vi "Drive PID.vi"(4 "reinitialize? (F)":bool, 6 "PID Params":T1={"PID gains"={"proportional gain (Kc)"=1.0, "integral time (Ti, min)"=0.0, "derivative time (Td, min)"=0.0}, "output range"={"output high"=1.0, "output low"=-1.0}}, 7 "Setpoint":dbl, 8 "Max Stop Speed":dbl, 9 "Distance Stop Threshold":dbl, 10 "Current Speed":dbl, 11 "Current Distance":dbl format="%#_13g") -> (0 "Finished":bool, 2 "output":dbl format="%.2f")   [LabVIEW 2014]
uses:
  <vilib>/addons/control/pid/pid.llb/PID (DBL).vi
  <vilib>/addons/control/pid/NI_PID_pid.lvlib
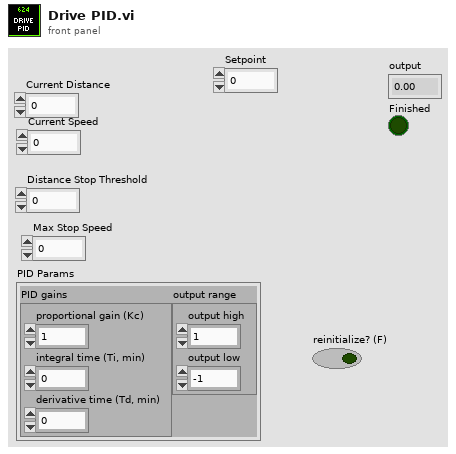
[diagram p1: front panel]
types:
  T1 = cluster{"PID gains":cluster{"proportional gain (Kc)":dbl, "integral time (Ti, min)":dbl, "derivative time (Td, min)":dbl}, "output range":cluster{"output high":dbl, "output low":dbl}}
  T2 = cluster{"proportional gain (Kc)":dbl, "integral time (Ti, min)":dbl, "derivative time (Td, min)":dbl}
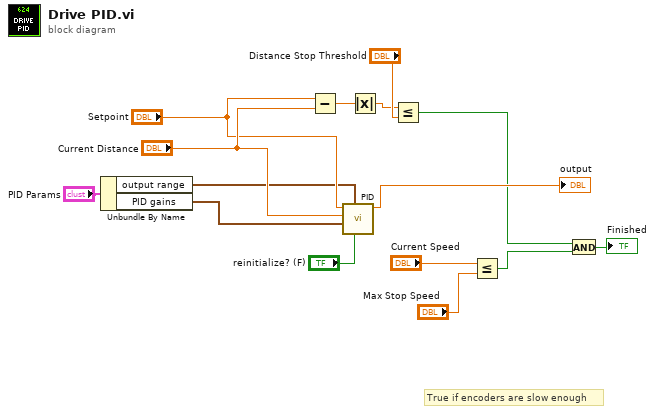
[diagram p0: block diagram]
diagram:
  # "True if encoders are slow enough"
  n1 = Unbundle By Name("PID Params") -> ("output range"=w12:cluster{"output high":dbl, "output low":dbl}, "PID gains"=w11:T2)
  n2 = Subtract(x="Setpoint", y="Current Distance") -> (x-y=w8:dbl)
  n3 = call-poly <vilib>:"PID.vi"("reinitialize? (F)"="reinitialize? (F)", "output range"=w12, "PID gains"=w11, "process variable"="Current Distance", "setpoint"="Setpoint") -> ("output"=→"output":dbl)  [unwired: 5 in, 1 out]
  n4 = Absolute Value(x=w8) -> (abs(x)=w6:dbl)
  n5 = Less Or Equal?(x=w6, y="Distance Stop Threshold") -> (x <= y?=w5:bool)
  n6 = Less Or Equal?(x="Current Speed", y="Max Stop Speed") -> (x <= y?=w2:bool)
  n7 = And(x=w5, y=w2) -> (x .and. y?=→"Finished":bool)
